vi "Initialize.vi"(8 "error in (no error)":errorcluster, 9 "Reset (True)":bool=TRUE, 10 "ID Query (True)":bool=TRUE, 11 "VISA resource name":refnum<visa-resource-name>) -> (0 "error out":errorcluster, 3 "VISA resource name out":refnum<visa-resource-name>)   [LabVIEW 2019, in "Tektronix AFG 3000 Series.lvlib"]
doc: "Establishes communication with the instrument and optionally performs an instrument identification query and/or an instrument reset. It also places the instrument in a default state needed for other instrument driver operations. Therefore, call this VI before calling other instrument driver VIs for this instrument. Generally, you need to call the <B>Initialize VI</B> only once at the beginning of an application."
uses:
  <userlib>/Tektronix AFG 3000 Series/Tektronix AFG 3000 Series.lvlib
panel:
  # "(c) 2006-2012 National Instruments.  ALL RIGHTS RESERVED."
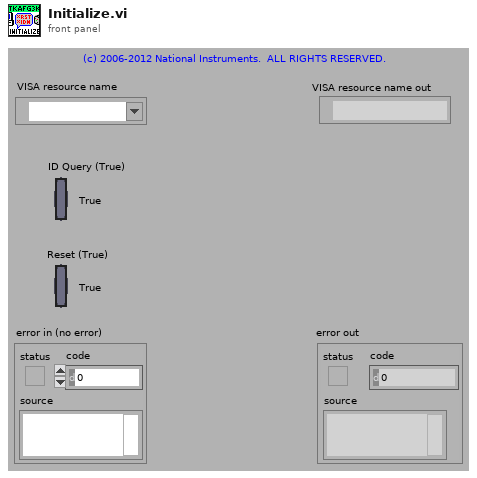
[diagram p1: front panel]
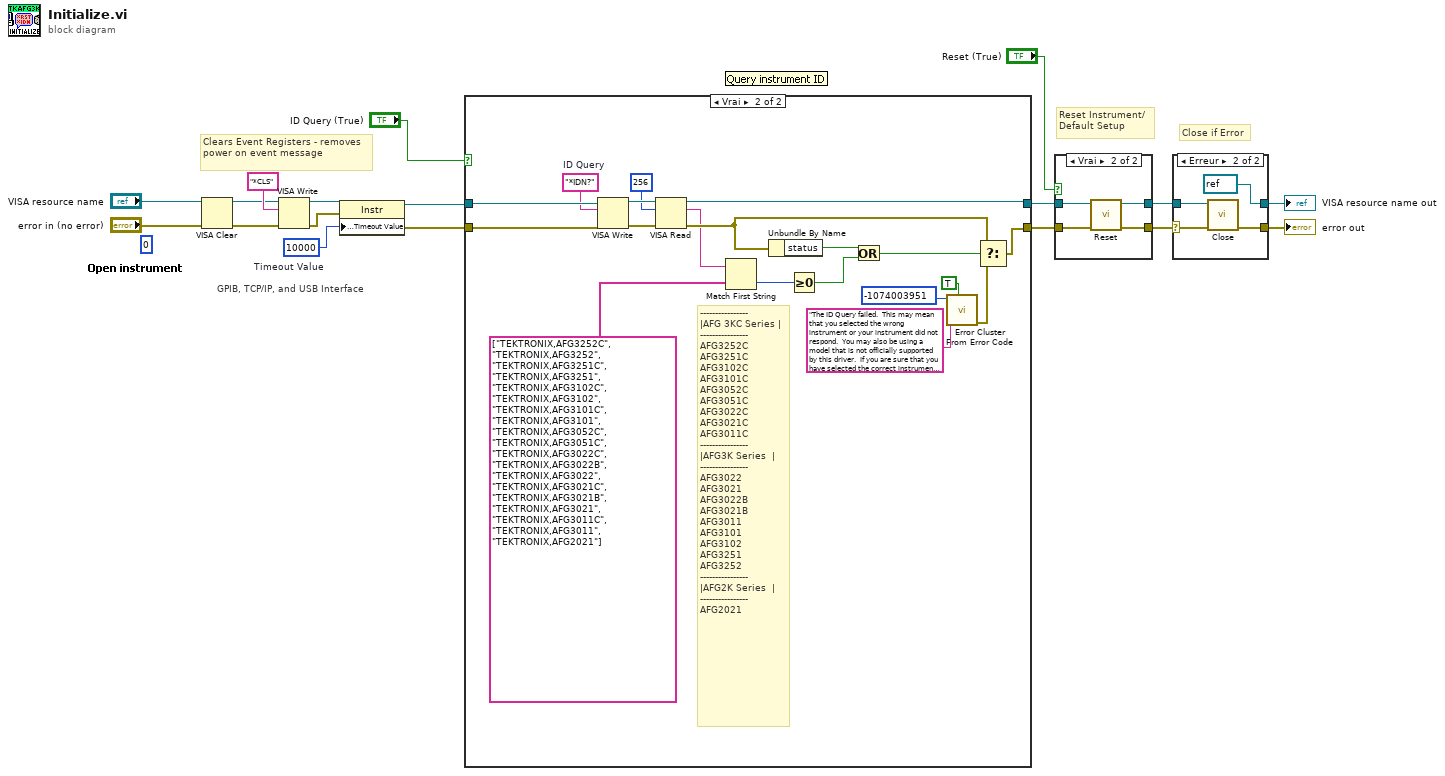
[diagram p0: block diagram]
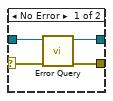
[diagram p2: hidden frame]
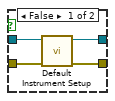
[diagram p3: hidden frame]
diagram:
  w8 = u32 10000  # Timeout Value
  (unwired) u32 0 ("access mode")
  # "Clears Event Registers - removes power on event message"
  # "GPIB, TCP/IP, and USB Interface"
  # "Close if Error"
  # "Reset Instrument/\nDefault Setup"
  n1 = VISA Clear(VISA resource name="VISA resource name", error in (no error)="error in (no error)") -> (VISA resource name out=w6:refnum<visa-resource-name>, error out=w5:errorcluster)
  n2 = VISA Write(VISA resource name=w6, write buffer="*CLS", error in (no error)=w5) -> (VISA resource name out=w4:refnum<visa-resource-name>, error out=w3:errorcluster)  [unwired: 1 out]
  n3 = property class="Instr"(reference=w4, error in=w3, "General Settings:Timeout Value"=w8) -> (reference out=w10:refnum<visa-resource-name>, error out=w9:errorcluster)
  n4 = case shown="Vrai" "ID Query (True)" {
    tunnel: [w19 w28] -> w11
    tunnel: [w20 w37] -> w12
    tunnel: w10 -> [w20 w38]
    tunnel: w9 -> [w19 w39]
    frame False {
    }
    frame True {
      w33 = "*IDN?"  # ID Query
      # "----------------\n|AFG 3KC Series |\n----------------\nAFG3252C\nAFG3251C\nAFG3102C\nAFG3101C\nAFG3052C\nAFG3051C\nAFG3022C\nAFG3021C\nAFG3011C\n----------------\n|AFG3K Series  |\n----------------\nAFG3022\nAFG3021\nAFG3022B\nAFG3021B\nAFG3011\nAFG3101\nAFG3102\nAFG3251\nAFG3252\n----------------\n|AFG2K Series  |\n----------------\nAFG2021"
      n5 = VISA Write(VISA resource name=w38, write buffer=w33, error in (no error)=w39) -> (VISA resource name out=w36:refnum<visa-resource-name>, error out=w35:errorcluster)  [unwired: 1 out]
      n6 = VISA Read(VISA resource name=w36, byte count=u32 256, error in (no error)=w35) -> (VISA resource name out=w37:refnum<visa-resource-name>, read buffer=w27:string, error out=w32:errorcluster)  [unwired: 1 out]
      n7 = Match First String(2:string[] ["TEKTRONIX,AFG3252C", "TEKTRONIX,AFG3252", "TEKTRONIX,AFG3251C", "TEKTRONIX,AFG3251", "TEKTRONIX,AFG3102C", "TEKTRONIX,AFG3102", "TEKTRONIX,AFG3101C", "TEKTRONIX,AFG3101", "TEKTRONIX,AFG3052C", "TEKTRONIX,AFG3051C", "TEKTRONIX,AFG3022C", "TEKTRONIX,AFG3022B", "TEKTRONIX,AFG3022", "TEKTRONIX,AFG3021C", "TEKTRONIX,AFG3021B", "TEKTRONIX,AFG3021", "TEKTRONIX,AFG3011C", "TEKTRONIX,AFG3011", "TEKTRONIX,AFG2021"] ("reversed array"), 3:w27) -> (0:w22:i32)  [unwired: 1 out]
      n8 = Unbundle By Name(w32) -> ("status"=w31:bool)
      n9 = Greater Or Equal To 0?(x=w22) -> (x >= 0?=w30:bool)
      n10 = Or(x=w31, y=w30) -> (x .or. y?=w29:bool)
      n11 = call <vilib>:"Error Cluster From Error Code.vi"("show call chain? (False)"=TRUE, "error message (\"\")"="The ID Query failed.  This may mean that you selected the wrong instrument or your instrument did not respond.  You may also be using a model that is not officially supported by this driver.  If you are sure that you have selected the correct instrument and it is responding, try disabling the ID Query." ("Source (VI Name)"), "error code (0)"=-1074003951 ("Code")) -> ("error out"=w23:errorcluster)  [unwired: 6 in]
      n12 = Select(t=w32, s=w29, f=w23) -> (s? t:f=w28:errorcluster)
    }
  }
  n13 = case shown="Vrai" "Reset (True)" {
    tunnel: [w42 w47] -> w13
    tunnel: w12 -> [w43 w45]
    tunnel: [w41 w46] -> w14
    tunnel: w11 -> [w40 w44]
    frame False {
      n14 = call <userlib>:"Default Instrument Setup.vi"("error in (no error)"=w40, "VISA resource name"=w43) -> ("error out"=w42:errorcluster, "VISA resource name out"=w41:refnum<visa-resource-name>)  [unwired: 8 in]
    }
    frame True {
      n15 = call <userlib>:"Reset.vi"("error in (no error)"=w44, "VISA resource name"=w45) -> ("error out"=w47:errorcluster, "VISA resource name out"=w46:refnum<visa-resource-name>)  [unwired: 8 in]
    }
  }
  n16 = case shown="Erreur" w13 {
    selector: w13 -> [w49 w53]
    tunnel: w14 -> [w48 w54]
    tunnel: [w51 refnum<visa-resource-name> refnum ("VISA resource name out")] -> w16
    tunnel: [w50 w55] -> w15
    frame No Error {
      n17 = call <userlib>:"Error Query.vi"("error in (no error)"=w49, "VISA resource name"=w48) -> ("error out"=w50:errorcluster, "VISA resource name out"=w51:refnum<visa-resource-name>)  [unwired: 6 in, 2 out]
    }
    frame Error {
      n18 = call <userlib>:"Close.vi"("error in (no error)"=w53, "VISA resource name"=w54) -> ("error out"=w55:errorcluster)  [unwired: 9 in]
    }
  }
  "VISA resource name out" <- w16
  "error out" <- w15
